vi "GDSLvIcon_SaveLayerInfo.vi"() -> ()   [LabVIEW 2020]
panel:
  in  "VI Ref in":refnum<vi>
  in  "error in (no error)":errorcluster
  out "VI Ref out":refnum<vi>
  out "error out":errorcluster
  in  "Data":string
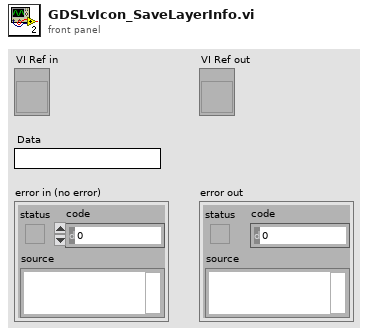
[diagram p1: front panel]
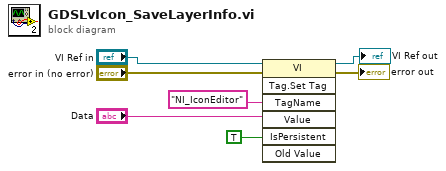
[diagram p0: block diagram]
diagram:
  n1 = invoke class="VI" method="Tag.Set Tag"(reference="VI Ref in", error in="error in (no error)", "TagName"="NI_IconEditor" ("Tag Name"), "Value"="Data", "IsPersistent"=TRUE ("Is Persistent")) -> (reference out=→"VI Ref out":refnum<vi>, error out=→"error out":errorcluster)  [unwired: 2 in, 5 out]
